vi "Initialise MAVLink.vi"() -> ()   [LabVIEW 2014]
uses:
  Global Variables/Global Variables.vi
  Controls/FGV Methods.ctl
panel:
  in  "Packet Sequence In":u8
  out "Initalize":u8(slide) scale=0.0..8.0
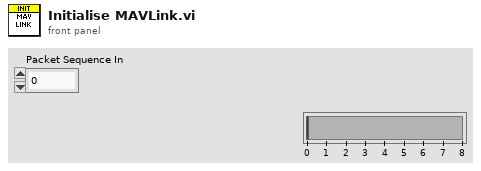
[diagram p1: front panel]
types:
  T1 = typedef "FGV Methods.ctl" = enum16{"Get", "Set"}
  T2 = cluster{"message_rate":u16, "stream_id":u8, "on_off":bool}
  T3 = cluster{"req_message_rate":u16, "target_system":u8, "target_component":u8, "req_stream_id":u8, "start_stop":bool}
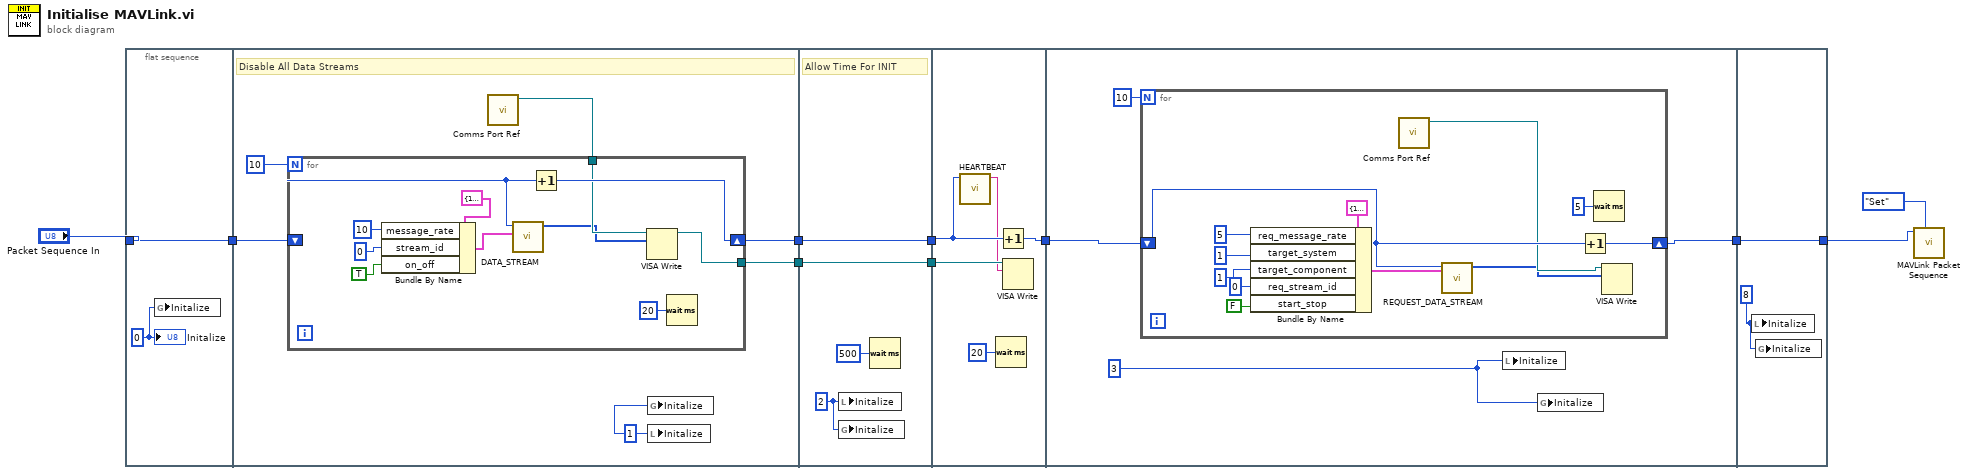
[diagram p0: block diagram]
diagram:
  n1 = flat-sequence {
    tunnel: "Packet Sequence In" -> [w12]
    tunnel: [w12] -> w5
    tunnel: [w17] -> w10
    tunnel: w5 -> [w18]
    tunnel: [w13] -> w2
    tunnel: w10 -> [w32]
    tunnel: [w32] -> w4
    tunnel: w2 -> [w30]
    tunnel: [w30] -> w1
    tunnel: w4 -> [w36]
    tunnel: [w37] -> w3
    tunnel: w1 -> [w38]
    tunnel: w3 -> [w42]
    tunnel: [w41] -> w6
    tunnel: [w56] -> w8
    tunnel: w6 -> [w56]
    frame #0 {
      w11 = u8 0 ("Initalize")
      n2 = global write "Global Variables.vi" "Initalize"(w11) -> ()
      "Initalize" <- w11
    }
    frame #1 {
      w15 = u8 1 ("Initalize")
      # "Disable All Data Streams"
      n3 = call "Comms Port Ref.vi"() -> ("Comms Port Ref"=w14:refnum<visa-resource-name>)  [unwired: 10 in, 1 out]
      n4 = for {
        N: 10 -> [_]
        shift-right: [w29] -> w17
        shift-left: w18 -> [w27]
        tunnel: w14 -> [w21]
        tunnel: [w19] -> w13
        n5 = Bundle By Name(cluster=T2 {"message_rate"=10, "stream_id"=0, "on_off"=FALSE} ("Payload"), "message_rate"=u16 10, "stream_id"=u8 0, "on_off"=TRUE) -> (w22:T2)
        n6 = call "DATA_STREAM.vi"("Payload"=w22, 11:w27) -> ("MAVLink Message"=w20:u8[])  [unwired: 9 in]
        n7 = Increment(x=w27) -> (x+1=w29:u8)
        n8 = VISA Write(VISA resource name=w21, write buffer=w20) -> (VISA resource name out=w19:refnum<visa-resource-name>)  [unwired: 1 in, 2 out]
        n9 = Wait (ms)(milliseconds to wait=u32 20) -> ()  [unwired: 1 out]
      }
      n10 = global write "Global Variables.vi" "Initalize"(w15) -> ()
      n11 = local write "Initalize"(w15) -> ()
    }
    frame #2 {
      w31 = u8 2 ("Initalize")
      # "Allow Time For INIT"
      n12 = local write "Initalize"(w31) -> ()
      n13 = global write "Global Variables.vi" "Initalize"(w31) -> ()
      n14 = Wait (ms)(milliseconds to wait=u32 500) -> ()  [unwired: 1 out]
    }
    frame #3 {
      n15 = call "HEARTBEAT.vi"("Packet Sequence"=w36) -> ("MAVLink MSG"=w35:string)  [unwired: 10 in]
      n16 = Wait (ms)(milliseconds to wait=u32 20) -> ()  [unwired: 1 out]
      n17 = Increment(x=w36) -> (x+1=w37:u8)
      n18 = VISA Write(VISA resource name=w38, write buffer=w35) -> ()  [unwired: 1 in, 3 out]
    }
    frame #4 {
      w40 = u8 3 ("Initalize")
      n19 = for {
        N: 10 -> [_]
        shift-right: [w53] -> w41
        shift-left: w42 -> [w54]
        n20 = Bundle By Name(cluster=T3 {"req_message_rate"=10, "target_system"=0, "target_component"=0, "req_stream_id"=0, "start_stop"=FALSE} ("Payload"), "req_message_rate"=u16 5, "target_system"=u8 1, "target_component"=u8 1, "req_stream_id"=u8 0, "start_stop"=FALSE) -> (w46:T3)
        n21 = call "Comms Port Ref.vi"() -> ("Comms Port Ref"=w52:refnum<visa-resource-name>)  [unwired: 10 in, 1 out]
        n22 = call "REQUEST_DATA_STREAM.vi"("Payload"=w46, 11:w54) -> ("MAVLink MSG"=w44:u8[])  [unwired: 9 in]
        n23 = Increment(x=w54) -> (x+1=w53:u8)
        n24 = Wait (ms)(milliseconds to wait=u32 5) -> ()  [unwired: 1 out]
        n25 = VISA Write(VISA resource name=w52, write buffer=w44) -> ()  [unwired: 1 in, 3 out]
      }
      n26 = local write "Initalize"(w40) -> ()
      n27 = global write "Global Variables.vi" "Initalize"(w40) -> ()
    }
    frame #5 {
      w55 = u8 8 ("Initalize")
      n28 = local write "Initalize"(w55) -> ()
      n29 = global write "Global Variables.vi" "Initalize"(w55) -> ()
    }
  }
  n30 = call "MAVLink Packet Sequence.vi"("FGV Method"=FGV_Methods."Set", "Packet Sequence In"=w8) -> ()  [unwired: 9 in, 1 out]
